vi "PrepareRollToPassRollerRole.vi"(6 "Tactic index in":i32, 7 "first call":bool, 8 "error in (no error)":errorcluster, 10 "Game in":refnum<class "Game.lvclass">, 11 "PrepareRollToPassRollerRole in":refnum<class "PrepareRollToPassRollerRole.lvclass">) -> (0 "error out":errorcluster, 1 "tactic index":i32, 2 "Robot out":refnum<class "Robot.lvclass">, 3 "PrepareRollToPassRollerRole out":refnum<class "PrepareRollToPassRollerRole.lvclass">)   [LabVIEW 2020, in "PrepareRollToPassRollerRole.lvclass"]
uses:
  PrepareRollToPassRollerRole.lvclass
  Robot_class/Robot.lvclass
  Game_class/Game.lvclass
  C:/Users/anton/Desktop/RoboIME/IC/SSL_AI/Role_class/Role.lvclass
  Role_class/Role.lvclass/Role.ctl
  PrepareRollToPassRollerRole.lvclass/PrepareRollToPassRollerRole.ctl
  Tacticbook_class/Tacticbook.lvclass/Tacticbook.ctl
  PrepareRollToPassRollerGoToTactic_class/PrepareRollToPassRollerGoToTactic.lvclass/PrepareRollToPassRollerGoToTactic.ctl
  RollerTactic_class/RollerTactic.lvclass/RollerTactic.ctl
  Tacticbook_class/Read PrepareRollToPassRollerGoToTactic.vi
  PrepareRollToPassRollerGoToTactic_class/Read States.vi
  Tacticbook_class/Write PrepareRollToPassRollerGoToTactic.vi
  Tacticbook_class/Read RollerTactic.vi
  RollerTactic_class/Read States.vi
  Tacticbook_class/Write RollerTactic.vi
  Role_class/Read Tacticbook.vi
  Read number_of_tactics.vi
  Role_class/Write Tacticbook.vi
  Role_class/Write tactic_index.vi
  Role_class/Read RobotRef.vi
  Tacticbook_class/Tacticbook.lvclass
  PrepareRollToPassRollerGoToTactic_class/PrepareRollToPassRollerGoToTactic.lvclass
  RollerTactic_class/RollerTactic.lvclass
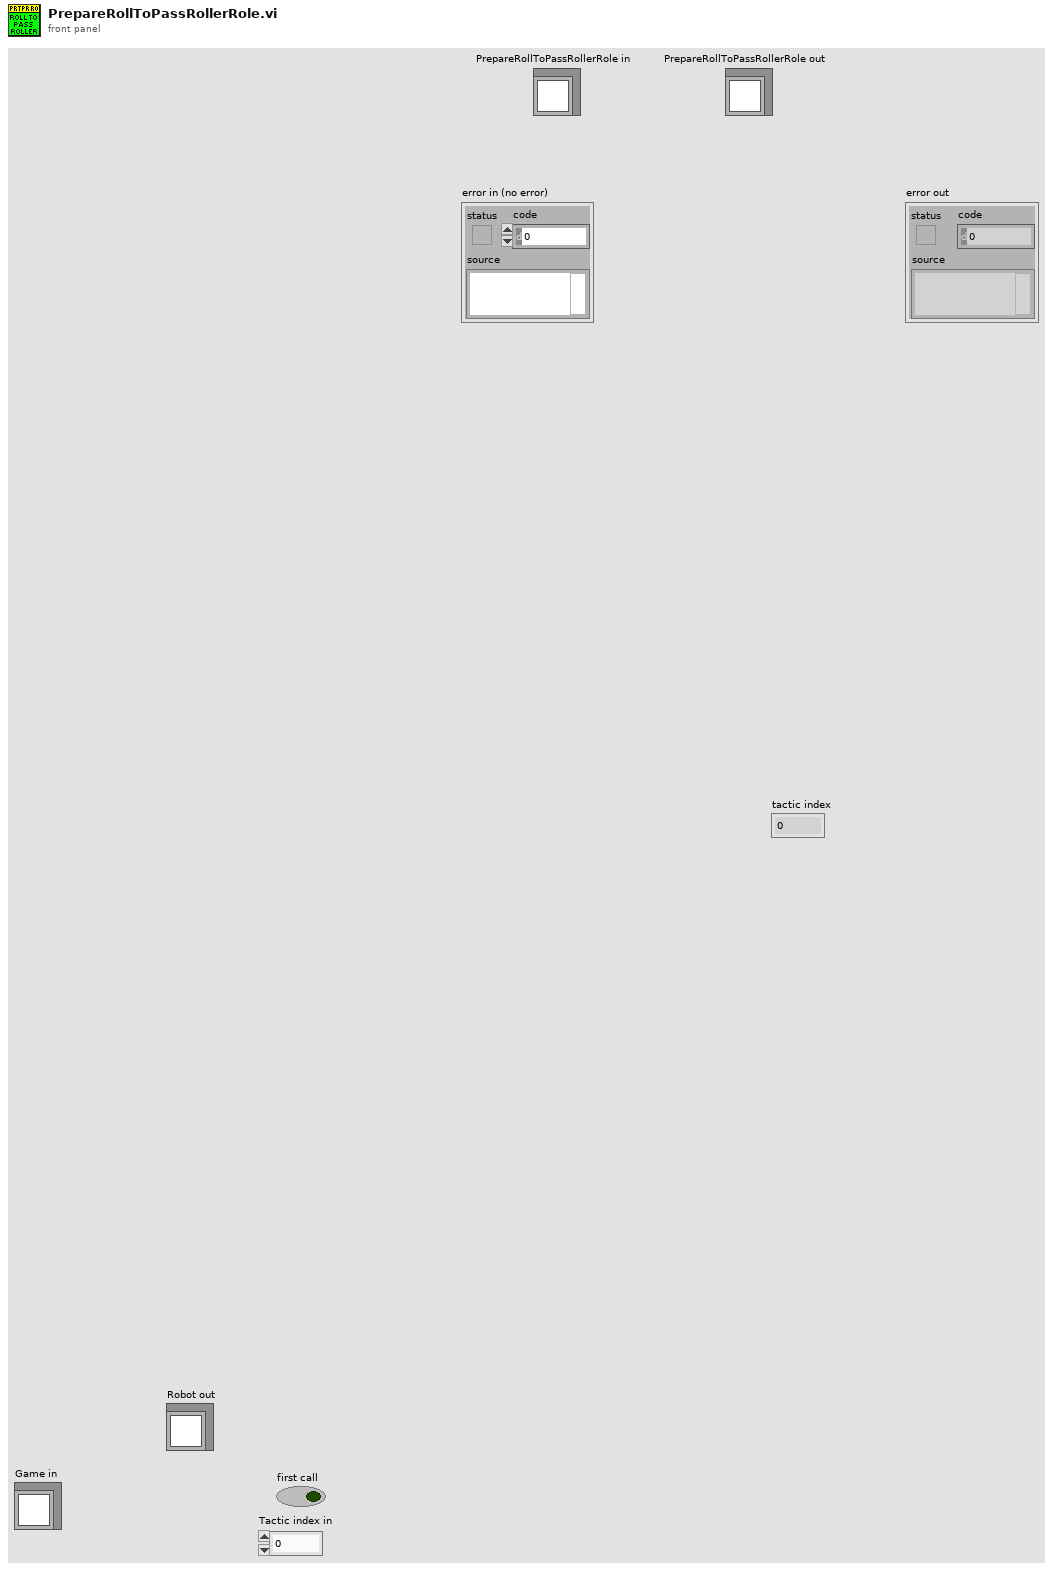
[diagram p1: front panel]
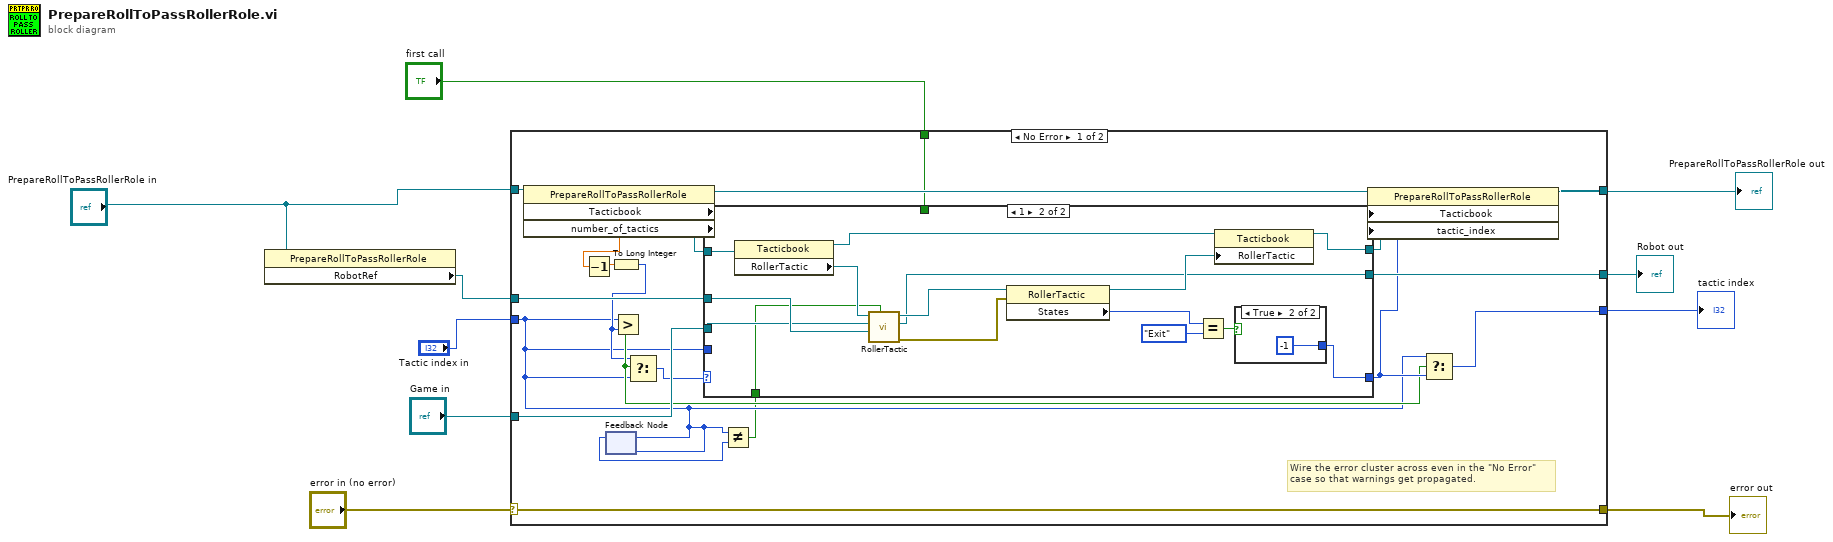
[diagram p0: block diagram]
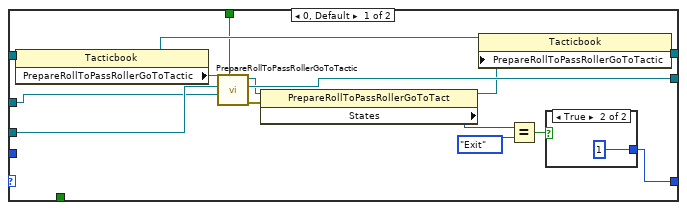
[diagram p2: hidden frame]
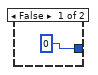
[diagram p3: hidden frame]
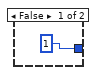
[diagram p4: hidden frame]
diagram:
  n1 = property class="PrepareRollToPassRollerRole"(reference="PrepareRollToPassRollerRole in") -> ("RobotRef"=w4:refnum<class "Robot.lvclass">)  [unwired: 1 in, 2 out]
  n2 = case shown="No Error" "error in (no error)" {
    selector: "error in (no error)" -> [w30 w67]
    tunnel: [w30 w67] -> w7
    tunnel: [w28 w66] -> w1
    tunnel: "PrepareRollToPassRollerRole in" -> [w29 w66]
    tunnel: w4 -> [w25 w65]
    tunnel: [w24 w65] -> w10
    tunnel: "Game in" -> [w22 _]
    tunnel: [w17 _] -> w6
    tunnel: "Tactic index in" -> [w12 _]
    tunnel: "first call" -> [w16 _]
    frame No Error {
      # "Wire the error cluster across even in the \"No Error\"\ncase so that warnings get propagated."
      n3 = property class="PrepareRollToPassRollerRole"(reference=w29) -> (reference out=w27:refnum<class "PrepareRollToPassRollerRole.lvclass">, "Tacticbook"=w26:refnum<class "Tacticbook.lvclass">, "number_of_tactics"=w21:dbl)  [unwired: 1 in, 1 out]
      n4 = Decrement(x=w21) -> (x-1=w14:dbl)
      n5 = feedback-in #1(w12) -> ()
      n6 = feedback #1(w12) -> (w13:i32)
      n7 = To Long Integer(number=w14) -> (32bit integer=w15:i32)
      n8 = Greater?(x=w12, y=w15) -> (0:w18:bool)
      n9 = Select(t=w15, s=w18, f=w12) -> (s? t:f=w20:i32)
      n10 = Not Equal?(x=w12, y=w13) -> (x != y?=w11:bool)
      n11 = case shown="1" w20 {
        tunnel: [w33 w50] -> w19
        tunnel: w26 -> [w45 w58]
        tunnel: w25 -> [w36 w53]
        tunnel: [w44 w55] -> w24
        tunnel: [w40 w54] -> w23
        tunnel: w22 -> [w37 w52]
        tunnel: w12 -> [_ _]
        tunnel: w16 -> [w32 _]
        tunnel: w11 -> [_ w48]
        frame 0, Default {
          n12 = property class="Tacticbook"(reference=w45) -> (reference out=w42:refnum<class "Tacticbook.lvclass">, "PrepareRollToPassRollerGoToTactic"=w39:refnum<class "PrepareRollToPassRollerGoToTactic.lvclass">)  [unwired: 1 in, 1 out]
          n13 = call "PrepareRollToPassRollerGoToTactic.vi"("first call"=w32, "Robot"=w36, "Game in"=w37, "PrepareRollToPassRollerGoToTactic in"=w39) -> ("error out"=w43:errorcluster, "Robot out"=w44:refnum<class "Robot.lvclass">, "PrepareRollToPassRollerGoToTactic out"=w38:refnum<class "PrepareRollToPassRollerGoToTactic.lvclass">)  [unwired: 5 in]
          n14 = property class="PrepareRollToPassRollerGoToTact"(reference=w38, error in=w43) -> (reference out=w41:refnum<class "PrepareRollToPassRollerGoToTactic.lvclass">, "States"=w34:enum16{"GoTo", "Exit"})  [unwired: 1 out]
          n15 = property class="Tacticbook"(reference=w42, "PrepareRollToPassRollerGoToTactic"=w41) -> (reference out=w40:refnum<class "Tacticbook.lvclass">)  [unwired: 1 in, 1 out]
          n16 = Equal?(x=w34, y=enum16{"GoTo", "Exit"}."Exit") -> (x = y?=w35:bool)
          n17 = case shown="True" w35 {
            tunnel: [0 1] -> w33
            frame False {
            }
            frame True {
            }
          }
        }
        frame 1 {
          n18 = property class="Tacticbook"(reference=w58) -> (reference out=w62:refnum<class "Tacticbook.lvclass">, "RollerTactic"=w57:refnum<class "RollerTactic.lvclass">)  [unwired: 1 in, 1 out]
          n19 = call "RollerTactic.vi"("first call"=w48, "Robot"=w53, "Game in"=w52, "RollerTactic in"=w57) -> ("error out"=w51:errorcluster, "Robot out"=w55:refnum<class "Robot.lvclass">, "RollerTactic out"=w56:refnum<class "RollerTactic.lvclass">)  [unwired: 5 in]
          n20 = property class="RollerTactic"(reference=w56, error in=w51) -> (reference out=w61:refnum<class "RollerTactic.lvclass">, "States"=w59:enum16{"Exit", "Roller"})  [unwired: 1 out]
          n21 = Equal?(x=w59, y=enum16{"Exit", "Roller"}."Exit") -> (x = y?=w60:bool)
          n22 = property class="Tacticbook"(reference=w62, "RollerTactic"=w61) -> (reference out=w54:refnum<class "Tacticbook.lvclass">)  [unwired: 1 in, 1 out]
          n23 = case shown="True" w60 {
            tunnel: [1 -1] -> w50
            frame False {
            }
            frame True {
            }
          }
        }
      }
      n24 = property class="PrepareRollToPassRollerRole"(reference=w27, "Tacticbook"=w23, "tactic_index"=w19) -> (reference out=w28:refnum<class "PrepareRollToPassRollerRole.lvclass">)  [unwired: 1 in, 1 out]
      n25 = Select(t=w12, s=w18, f=w19) -> (s? t:f=w17:i32)
    }
    frame Error {
    }
  }
  "error out" <- w7
  "Robot out" <- w10
  "tactic index" <- w6
  "PrepareRollToPassRollerRole out" <- w1
